vi "EOL CAN_Get_Motor_CycleCount_and_Mode.vi"(11 "NetworkObjHandle":T2) -> (0 "Controller Mode":T1, 1 "Slide Cycles":u16, 2 "Vent Cycles":u16, 3 "Response Good?":bool, 5 "TxRx Data":string[][](array[string]))   [LabVIEW 2018]
uses:
  <vilib>/nican/nican.llb/xobjhandle.ctl
  <userlib>/type defs/17x Motor Mode Control.ctl
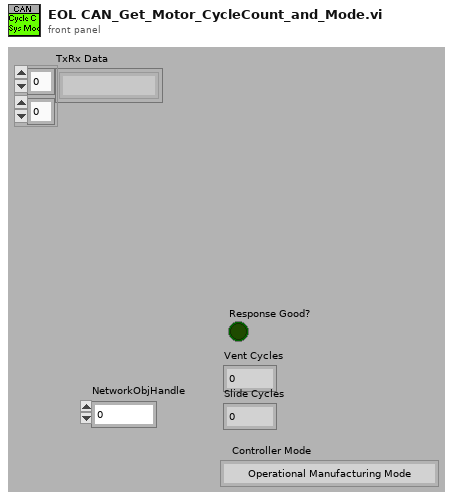
[diagram p1: front panel]
types:
  T1 = typedef "17x Motor Mode Control.ctl" = enum16{"Operational Manufacturing Mode", "Supervised Manufacturing Mode", "Slide Operational Manufacturing Mode", "Vent Operational Manufacturing Mode", "Operational User Mode", "Invalid Mode"}
  T2 = typedef "xobjhandle.ctl" = u32
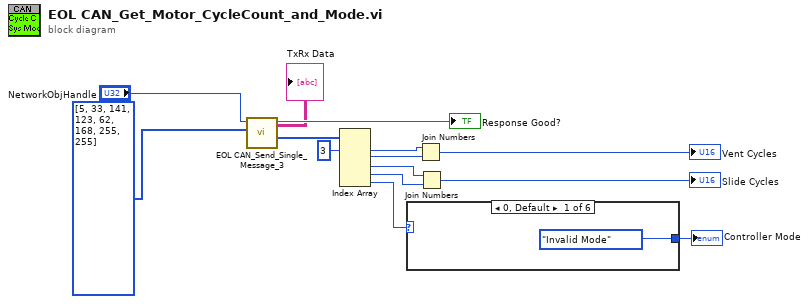
[diagram p0: block diagram]
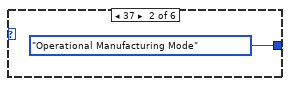
[diagram p2: hidden frame]
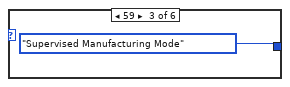
[diagram p3: hidden frame]
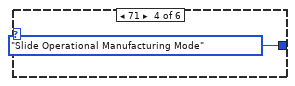
[diagram p4: hidden frame]
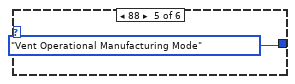
[diagram p5: hidden frame]
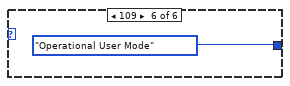
[diagram p6: hidden frame]
diagram:
  n1 = call <userlib>:"EOL CAN_Send_Single_Message_3.vi"("Tx Msg"=u8[] [5, 33, 141, 123, 62, 168, 255, 255] ("Transmit Data"), "NetworkObjHandle"="NetworkObjHandle") -> ("Rx Message"=w2:u8[], "Response Good?"=→"Response Good?":bool, "TxRx Data"=→"TxRx Data":string[][])  [unwired: 6 in, 1 out]
  n2 = Index Array(array=w2, index #1=3 ("index")) -> (element #1=w4:u8, element #2=w5:u8, element #3=w6:u8, element #4=w7:u8, element #5=w10:u8)  [unwired: 4 in]
  n3 = case shown="0, Default" w10 {
    tunnel: [17x_Motor_Mode_Control."Invalid Mode" ("Controller Mode 2") 17x_Motor_Mode_Control."Operational Manufacturing Mode" ("Controller Mode 2") 17x_Motor_Mode_Control."Supervised Manufacturing Mode" ("Controller Mode 2") 17x_Motor_Mode_Control."Slide Operational Manufacturing Mode" ("Controller Mode 2") 17x_Motor_Mode_Control."Vent Operational Manufacturing Mode" ("Controller Mode 2") 17x_Motor_Mode_Control."Operational User Mode" ("Controller Mode 2")] -> w11
    frame 0, Default {
    }
    frame 37 {
    }
    frame 59 {
    }
    frame 71 {
    }
    frame 88 {
    }
    frame 109 {
    }
  }
  "Controller Mode" <- w11
  n4 = Join Numbers(hi=w4, lo=w5) -> ((hi.lo)=→"Vent Cycles":u16)
  n5 = Join Numbers(hi=w6, lo=w7) -> ((hi.lo)=→"Slide Cycles":u16)
